vi "Keithley2420subVI_V2.vi"(11 "K-2420 init":T1) -> (1 "String":string, 2 "Resistance":sgl, 3 "Cluster":T1)   [LabVIEW 2014]
uses:
  Drivers and Software/LabVIEW 8.2 Drivers/keithley_24xx/Keithley 24XX/Public/Data/Read (Single Point).vi
  Drivers and Software/keithley_24xx/Keithley 24XX/Keithley 24XX.lvlib
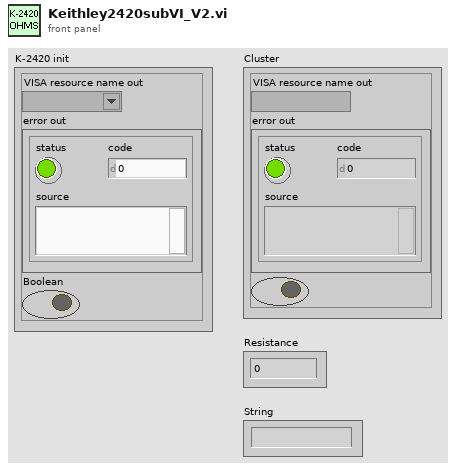
[diagram p1: front panel]
types:
  T1 = cluster{"VISA resource name out":refnum<visa-resource-name>, "error out":errorcluster, "Boolean":bool}
  T2 = cluster{"VISA resource name out":refnum<visa-resource-name>, "error out":errorcluster, bool}
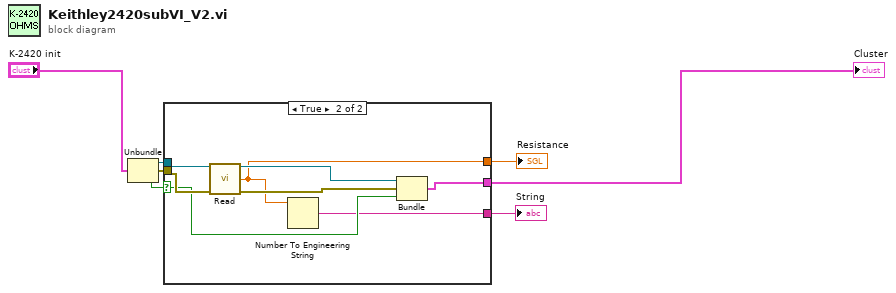
[diagram p0: block diagram]
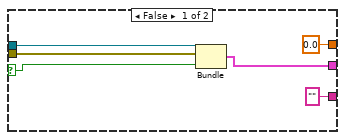
[diagram p2: hidden frame]
diagram:
  n1 = Unbundle("K-2420 init") -> ("VISA resource name out"=w2:refnum<visa-resource-name>, "error out"=w3:errorcluster, "Boolean"=w4:bool)
  n2 = case shown="True" w4 {
    selector: w4 -> [w11 w17]
    tunnel: w2 -> [w13 w19]
    tunnel: w3 -> [w12 w18]
    tunnel: [w10 w16] -> w7
    tunnel: ["" w15] -> w5
    tunnel: [sgl 0.0 ("Resistance") w14] -> w6
    frame False {
      n3 = Bundle("VISA resource name out"=w13, "error out"=w12, w11) -> (w10:T2)  [unwired: 1 in]
    }
    frame True {
      n4 = call-poly "Read.vi"("VISA resource name"=w19, "error in (no error)"=w18) -> ("VISA resource name out"=w20:refnum<visa-resource-name>, "Resistance"=w14:sgl, "error out"=w21:errorcluster)  [unwired: 7 in, 4 out]
      n5 = Number To Engineering String(4:w14) -> (0:w15:string)  [unwired: 3 in]
      n6 = Bundle("VISA resource name out"=w20, "error out"=w21, w17) -> (w16:T2)  [unwired: 1 in]
    }
  }
  "Cluster" <- w7
  "Resistance" <- w6
  "String" <- w5
